vi "PIM Determine Channel Type From Name.vi"(10 "Channel Name":string) -> (2 "Channel Type":T1)   [LabVIEW 2011]
uses:
  TypeDefs/PIM Channel Type.ctl
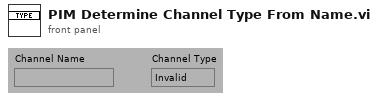
[diagram p1: front panel]
types:
  T1 = typedef "PIM Channel Type.ctl" = enum16{"Invalid", "Frequency", "Power", "CheckTx", "Unleveled", "Squelch", "Time", "Ref Limit", "IM Overload", "IM Power", "IM Frequency"}
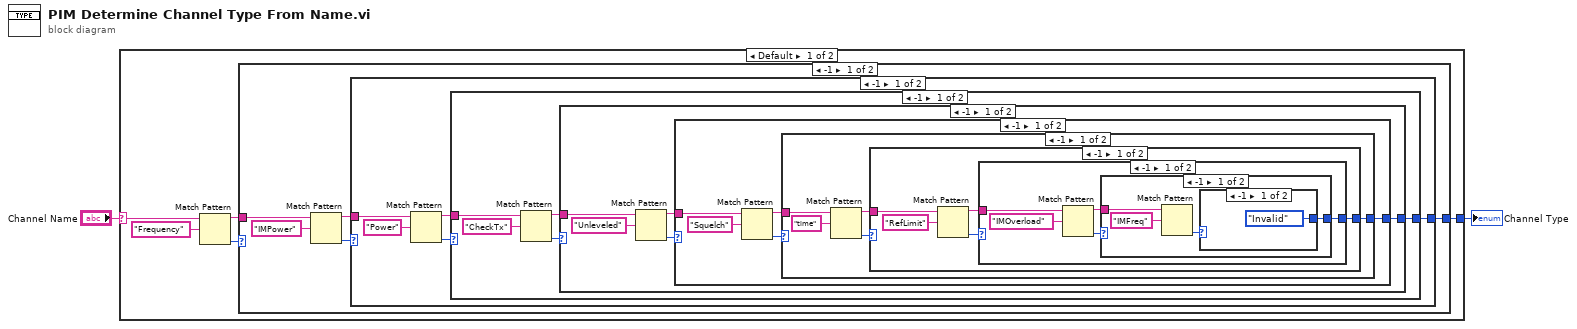
[diagram p0: block diagram]
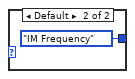
[diagram p2: hidden frame]
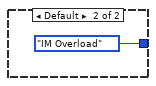
[diagram p3: hidden frame]
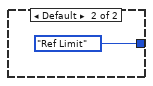
[diagram p4: hidden frame]
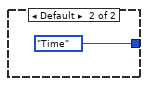
[diagram p5: hidden frame]
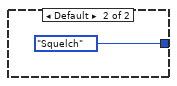
[diagram p6: hidden frame]
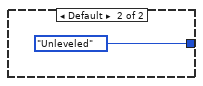
[diagram p7: hidden frame]
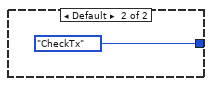
[diagram p8: hidden frame]
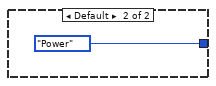
[diagram p9: hidden frame]
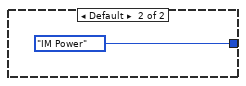
[diagram p10: hidden frame]
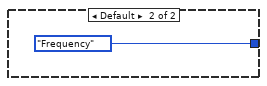
[diagram p11: hidden frame]
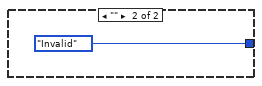
[diagram p12: hidden frame]
diagram:
  n1 = case shown="Default" "Channel Name" {
    selector: "Channel Name" -> [w4 _]
    tunnel: [w5 PIM_Channel_Type."Invalid" ("Channel Type")] -> w2
    frame Default {
      n2 = Match Pattern(string=w4, regular expression="Frequency") -> (before substring=w3:string, offset past match=w6:i32)  [unwired: 3 out]
      n3 = case shown="-1" w6 {
        tunnel: [w12 PIM_Channel_Type."Frequency" ("Channel Type")] -> w5
        tunnel: w3 -> [w10 _]
        frame -1 {
          n4 = Match Pattern(string=w10, regular expression="IMPower") -> (before substring=w8:string, offset past match=w9:i32)  [unwired: 3 out]
          n5 = case shown="-1" w9 {
            tunnel: [w17 PIM_Channel_Type."IM Power" ("Channel Type")] -> w12
            tunnel: w8 -> [w15 _]
            frame -1 {
              n6 = Match Pattern(string=w15, regular expression="Power") -> (before substring=w13:string, offset past match=w14:i32)  [unwired: 3 out]
              n7 = case shown="-1" w14 {
                tunnel: [w22 PIM_Channel_Type."Power" ("Channel Type")] -> w17
                tunnel: w13 -> [w20 _]
                frame -1 {
                  n8 = Match Pattern(string=w20, regular expression="CheckTx") -> (before substring=w18:string, offset past match=w19:i32)  [unwired: 3 out]
                  n9 = case shown="-1" w19 {
                    tunnel: [w26 PIM_Channel_Type."CheckTx" ("Channel Type")] -> w22
                    tunnel: w18 -> [w25 _]
                    frame -1 {
                      n10 = Match Pattern(string=w25, regular expression="Unleveled") -> (before substring=w23:string, offset past match=w24:i32)  [unwired: 3 out]
                      n11 = case shown="-1" w24 {
                        tunnel: [w32 PIM_Channel_Type."Unleveled" ("Channel Type")] -> w26
                        tunnel: w23 -> [w30 _]
                        frame -1 {
                          n12 = Match Pattern(string=w30, regular expression="Squelch") -> (before substring=w28:string, offset past match=w29:i32)  [unwired: 3 out]
                          n13 = case shown="-1" w29 {
                            tunnel: [w37 PIM_Channel_Type."Squelch" ("Channel Type")] -> w32
                            tunnel: w28 -> [w35 _]
                            frame -1 {
                              n14 = Match Pattern(string=w35, regular expression="time") -> (before substring=w33:string, offset past match=w34:i32)  [unwired: 3 out]
                              n15 = case shown="-1" w34 {
                                tunnel: [w42 PIM_Channel_Type."Time" ("Channel Type")] -> w37
                                tunnel: w33 -> [w40 _]
                                frame -1 {
                                n16 = Match Pattern(string=w40, regular expression="RefLimit") -> (before substring=w38:string, offset past match=w39:i32)  [unwired: 3 out]
                                n17 = case shown="-1" w39 {
                                tunnel: [w47 PIM_Channel_Type."Ref Limit" ("Channel Type")] -> w42
                                tunnel: w38 -> [w45 _]
                                frame -1 {
                                n18 = Match Pattern(string=w45, regular expression="IMOverload") -> (before substring=w43:string, offset past match=w44:i32)  [unwired: 3 out]
                                n19 = case shown="-1" w44 {
                                tunnel: [w49 PIM_Channel_Type."IM Overload" ("Channel Type")] -> w47
                                tunnel: w43 -> [w50 _]
                                frame -1 {
                                n20 = Match Pattern(string=w50, regular expression="IMFreq") -> (offset past match=w48:i32)  [unwired: 4 out]
                                n21 = case shown="-1" w48 {
                                tunnel: [PIM_Channel_Type."Invalid" ("Channel Type") PIM_Channel_Type."IM Frequency" ("Channel Type")] -> w49
                                frame -1 {
                                }
                                frame Default {
                                }
                                }
                                }
                                frame Default {
                                }
                                }
                                }
                                frame Default {
                                }
                                }
                                }
                                frame Default {
                                }
                              }
                            }
                            frame Default {
                            }
                          }
                        }
                        frame Default {
                        }
                      }
                    }
                    frame Default {
                    }
                  }
                }
                frame Default {
                }
              }
            }
            frame Default {
            }
          }
        }
        frame Default {
        }
      }
    }
    frame "" {
    }
  }
  "Channel Type" <- w2
